vi "Calculate heading.vi"(10 "Y array":dbl[](array[numeric]), 11 "X array":dbl[](array[numeric])) -> (0 "Closest obstacle (y)":dbl, 1 "Closest obstacle (x)":dbl, 2 "Turn in place":bool, 3 "Heading":dbl)   [LabVIEW 2010]
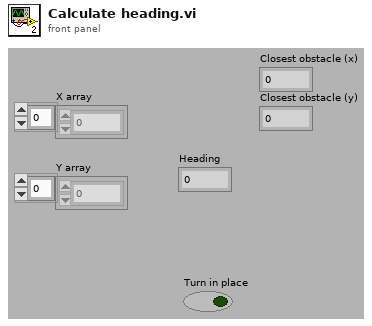
[diagram p1: front panel]
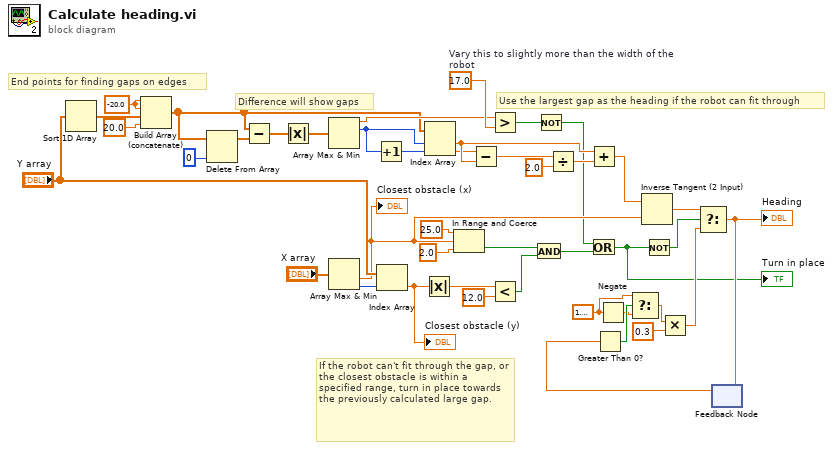
[diagram p0: block diagram]
diagram:
  w18 = 1.5707963267948966
  w34 = 17.0  # Vary this to slightly more than the width of the robot
  w32 = -20.0 ("element")
  # "If the robot can't fit through the gap, or the closest obstacle is within a specified range, turn in place towards the previously calculated large gap."
  # "End points for finding gaps on edges"
  # "Use the largest gap as the heading if the robot can fit through"
  # "Difference will show gaps"
  n1 = Sort 1D Array(array="Y array") -> (sorted array=w42:dbl[])
  n2 = Build Array (concatenate)(w32, w32, w42, 20.0 ("element")) -> (w29:dbl[])
  n3 = Delete From Array(array=w29, index=0) -> (array with subset deleted=w25:dbl[])  [unwired: 1 in, 1 out]
  n4 = Subtract(x=w29, y=w25) -> (x-y=w24:dbl[])
  n5 = Absolute Value(x=w24) -> (abs(x)=w28:dbl[])
  n6 = Array Max & Min(array=w28) -> (max value=w33:dbl, max index (indices)=w30:i32)  [unwired: 2 out]
  n7 = Array Max & Min(array="X array") -> (min value=w4:dbl, min index (indices)=w13:i32)  [unwired: 2 out]
  "Closest obstacle (x)" <- w4
  n8 = Increment(x=w30) -> (x+1=w31:i32)
  n9 = Index Array(array="Y array", index=w13) -> (element=w5:dbl)
  "Closest obstacle (y)" <- w5
  n10 = Absolute Value(x=w5) -> (abs(x)=w12:dbl)
  n11 = Index Array(array=w29, index #1=w30, index #2=w31) -> (element #1=w39:dbl, element #2=w35:dbl)
  n12 = In Range and Coerce(upper limit=25.0 ("y"), x=w4, lower limit=2.0) -> (In Range?=w6:bool)  [unwired: 1 out]
  n13 = Subtract(x=w35, y=w39) -> (x-y=w36:dbl)
  n14 = Greater?(x=w33, y=w34) -> (0:w23:bool)
  n15 = Less?(x=w12, y=12.0) -> (x < y?=w10:bool)
  n16 = And(x=w6, y=w10) -> (x .and. y?=w9:bool)
  n17 = Not(x=w23) -> (.not. x?=w3:bool)
  n18 = Divide(x=w36, y=2.0) -> (x/y=w38:dbl)
  n19 = Add(x=w39, y=w38) -> (x+y=w40:dbl)
  n20 = Or(x=w3, y=w9) -> (x .or. y?=w2:bool)
  "Turn in place" <- w2
  n21 = Negate(x=w18) -> (-x=w17:dbl)
  n22 = Inverse Tangent (2 Input)(1:w4, 2:w40) -> (0:w41:dbl)
  n23 = Not(x=w2) -> (.not. x?=w1:bool)
  n24 = feedback #1() -> (w21:dbl)  [unwired: 1 in]
  n25 = Greater Than 0?(x=w21) -> (x > 0?=w20:bool)
  n26 = Select(t=w18, s=w20, f=w17) -> (s? t:f=w19:dbl)
  n27 = Multiply(x=w19, y=0.3) -> (x*y=w16:dbl)
  n28 = Select(t=w41, s=w1, f=w16) -> (s? t:f=w22:dbl)
  "Heading" <- w22
  n29 = feedback-in #1(w22) -> ()
